vi "ROI_to_Mask_Error_Free.vi"(8 "error in (no error)":errorcluster, 9 "Image Size":cluster{"X":i32, "Y":i32}={"X"=640, "Y"=480}, 10 "ROI in":T2, 11 "Refnum in":T1) -> (0 "error out":errorcluster, 2 "ROI out":T3, 3 "Refnum out":T1)   [LabVIEW 2019]
uses:
  <vilib>/vision/Image Controls.llb/IMAQ Image.ctl
  <vilib>/vision/NI_Vision_Development_Module.lvlib
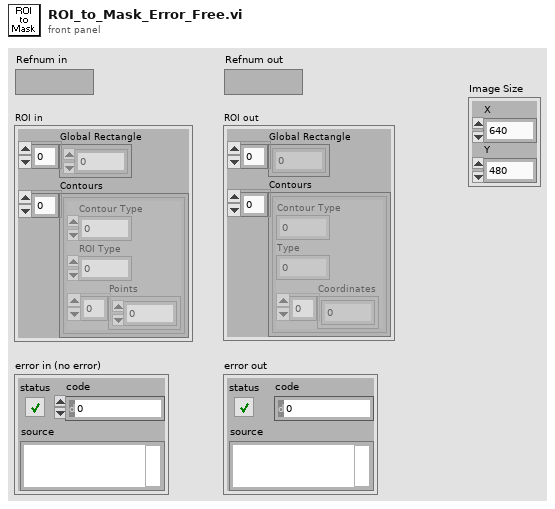
[diagram p1: front panel]
types:
  T1 = typedef "IMAQ Image.ctl" = refnum<image>
  T2 = cluster{"Global Rectangle":i32[], "Contours":cluster{"Contour Type":u32, "ROI Type":u32, "Points":i32[]}[]}
  T3 = cluster{"Global Rectangle":i32[], "Contours":cluster{"Contour Type":u32, "Type":u32, "Coordinates":i32[]}[]}
  T4 = typedef "IMAQ Rectangle" = cluster{"Left":i32, "Top":i32, "Right":i32, "Bottom":i32, "Rotation":dbl}
  T5 = typedef "ROI Descriptor" = cluster{"Global Rectangle":i32[], "Contours":cluster{"ID":enum32{"External", "Internal"}, "Type":u32, "Coordinates":i32[]}[]}
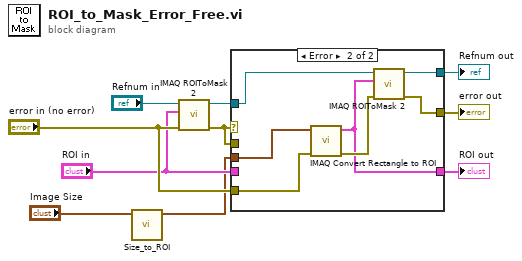
[diagram p0: block diagram]
diagram:
  n1 = call "Size_to_ROI.vi"("Image Size"="Image Size") -> ("Rectangle"=w1:T4)  [unwired: 10 in]
  n2 = call "IMAQ ROIToMask 2"("error in (no error)"="error in (no error)", "ROI Descriptor"="ROI in", "Image"="Refnum in") -> ("error out"=w8:errorcluster, "Image Out"=w7:T1)  [unwired: 6 in, 1 out]
  n3 = case shown="Error" w8 {
    tunnel: w8 -> [w13 _]
    tunnel: [w13 w15] -> w3
    tunnel: "error in (no error)" -> [_ w20]
    tunnel: [w12 w17] -> w6
    tunnel: "ROI in" -> [w12 _]
    tunnel: w7 -> [w11 w18]
    tunnel: [w11 w16] -> w10
    tunnel: w1 -> [_ w14]
    frame No Error {
    }
    frame Error {
      n4 = call "IMAQ Convert Rectangle to ROI"("error in (no error)"=w20, "Rectangle"=w14) -> ("error out"=w19:errorcluster, "ROI Descriptor"=w17:T5)  [unwired: 7 in]
      n5 = call "IMAQ ROIToMask 2"("error in (no error)"=w19, "ROI Descriptor"=w17, "Image"=w18) -> ("error out"=w15:errorcluster, "Image Out"=w16:T1)  [unwired: 6 in, 1 out]
    }
  }
  "Refnum out" <- w10
  "ROI out" <- w6
  "error out" <- w3
